vi "Source Off Limit Voltage.vi"(7 "Voltage Limit (40)":dbl=40.0, 8 "error in (no error)":errorcluster, 9 "Channel (Channel A)":T1, 10 "Node In":string, 11 "VISA resource name":refnum<visa-resource-name>) -> (0 "error out":errorcluster, 1 "Command String":string, 2 "Node Out":string, 3 "VISA resource name out":refnum<visa-resource-name>)   [LabVIEW 2018, in "Keithley 2600 Series.lvlib"]
doc: "This attribute sets the limit used when the source-measure unit is in normal output-off mode, the output is off, and the smuX.source.offfunc is set to smuX.OUTPUT_DCAMPS. \n\n<b>Functions and Attributes Used</b>\nsmuX.source.offlimitv"
uses:
  Keithley 2600 Series.lvlib
  Private/GlobalVariables.vi
  Channel.ctl
panel:
  # "(c) 2011 Keithley Instruments, Inc.  ALL RIGHTS RESERVED."
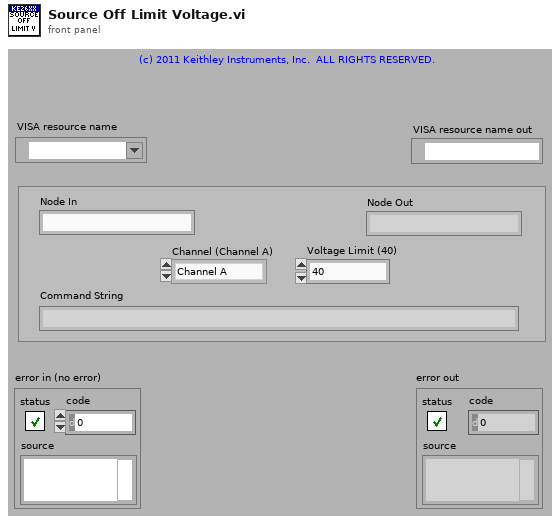
[diagram p1: front panel]
types:
  T1 = typedef "Keithley 2600 Series.lvlib/Channel.ctl" = enum32{"Channel A", "Channel B"}
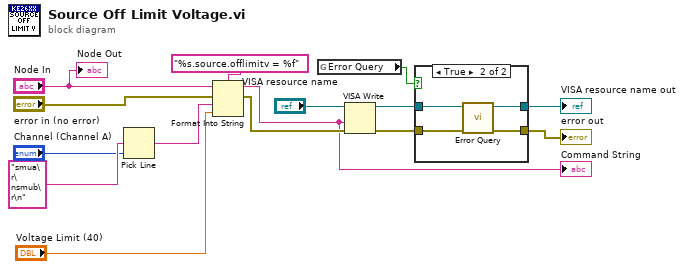
[diagram p0: block diagram]
diagram:
  n1 = Pick Line(multi-line string="smua\r\nsmub\r\n" ("options"), line index="Channel (Channel A)") -> (output string=w5:string)  [unwired: 1 out]
  n2 = Format Into String(format string="%s.source.offlimitv = %f", initial string="Node In", error in="error in (no error)", w5, "Voltage Limit (40)") -> (resulting string=w2:string, error out=w3:errorcluster)
  "Command String" <- w2
  n3 = global read "GlobalVariables.vi" "Error Query"() -> (w13:bool)
  n4 = VISA Write(VISA resource name="VISA resource name", write buffer=w2, error in (no error)=w3) -> (VISA resource name out=w12:refnum<visa-resource-name>, error out=w11:errorcluster)  [unwired: 1 out]
  n5 = case shown="True" w13 {
    tunnel: w12 -> [w17 w21]
    tunnel: w11 -> [w16 w20]
    tunnel: [w17 w19] -> w10
    tunnel: [w16 w18] -> w9
    frame False {
    }
    frame True {
      n6 = call "Error Query.vi"("error in (no error)"=w20, "VISA resource name"=w21) -> ("error out"=w18:errorcluster, "VISA resource name out"=w19:refnum<visa-resource-name>)  [unwired: 8 out]
    }
  }
  "VISA resource name out" <- w10
  "error out" <- w9
  "Node Out" <- "Node In"
